vi "RSZVB Set Mixer Delay Measurement Setup.vi"(8 "error in (no error)":errorcluster {"code" format="%.0x"}, 9 "Measurement Setup (Internal Receiver)":i32(ring) items=["Internal Receiver", "External Receiver"], 10 "Channel (1)":i32=1, 11 "VISA session":refnum<visa-resource-name>) -> (0 "error out":errorcluster {"code" format="%.0x"}, 3 "dup VISA session":refnum<visa-resource-name>)   [LabVIEW 2011]
doc: "Selects the measurement setup/receiver configuration for the mixer delay measurement. \n\nNotes:\n\n(1) This mode requires options R&S ZVA-K9 and R&S ZVA-K4\n\nRemote-control command(s):\n[SENSe<Ch>:]FREQuency:MDELay:RECeiver INTernal | EXTernal"
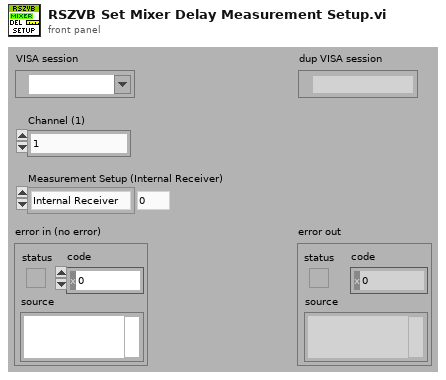
[diagram p1: front panel]
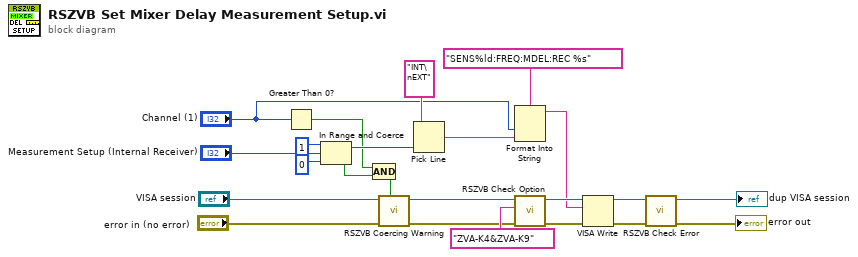
[diagram p0: block diagram]
diagram:
  n1 = Greater Than 0?(x="Channel (1)") -> (x > 0?=w11:bool)
  n2 = In Range and Coerce(upper limit=1, x="Measurement Setup (Internal Receiver)", lower limit=0) -> (coerced(x)=w14:i32, In Range?=w12:bool)
  n3 = Compound Arithmetic op=AND(w11, w12) -> (w10:bool)
  n4 = call "RSZVB Coercing Warning.vi"("In Range?"=w10, "error in (no error)"="error in (no error)", "VISA session"="VISA session") -> ("error out"=w3:errorcluster, "dup VISA session"=w4:refnum<visa-resource-name>)  [unwired: 7 in]
  n5 = Pick Line(multi-line string="INT\nEXT", line index=w14) -> (output string=w8:string)  [unwired: 1 in]
  n6 = Format Into String(format string="SENS%ld:FREQ:MDEL:REC %s", "Channel (1)", w8) -> (resulting string=w19:string)  [unwired: 2 in, 1 out]
  n7 = call "RSZVB Check Option.vi"("error in (no error)"=w3, "Options"="ZVA-K4&ZVA-K9", "VISA session"=w4) -> ("error out"=w21:errorcluster, "dup VISA session"=w20:refnum<visa-resource-name>)  [unwired: 7 in]
  n8 = VISA Write(VISA resource name=w20, write buffer=w19, error in (no error)=w21) -> (VISA resource name out=w17:refnum<visa-resource-name>, error out=w18:errorcluster)  [unwired: 1 out]
  n9 = call "RSZVB Check Error.vi"("error in (no error)"=w18, "VISA session"=w17) -> ("error out"=→"error out":errorcluster, "dup VISA session"=→"dup VISA session":refnum<visa-resource-name>)  [unwired: 8 in]
